vi "Read u.vi"(8 "error in (no error)":errorcluster, 11 "tCRD Data in":refnum<class "tCRD Data.lvclass">) -> (0 "error out":errorcluster, 2 "u":sgl, 3 "tCRD Data out":refnum<class "tCRD Data.lvclass">)   [LabVIEW 2013, in "tCRD Data.lvclass"]
uses:
  tCRD Data.lvclass
  tCRD Data.lvclass/tCRD Data.ctl
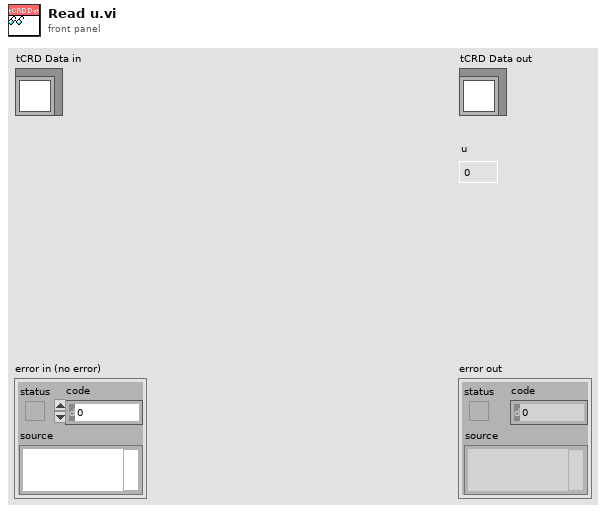
[diagram p1: front panel]
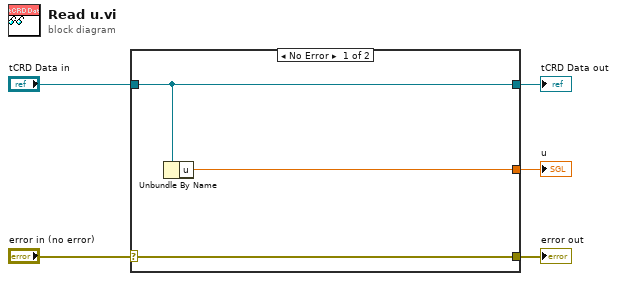
[diagram p0: block diagram]
diagram:
  n1 = case shown="No Error" "error in (no error)" {
    selector: "error in (no error)" -> [w8 w9]
    tunnel: [w8 w9] -> w4
    tunnel: [w7 w10] -> w2
    tunnel: "tCRD Data in" -> [w7 w10]
    tunnel: [w6 _] -> w1
    frame No Error {
      n2 = Unbundle By Name(w7) -> ("u"=w6:sgl)
    }
    frame Error {
    }
  }
  "error out" <- w4
  "tCRD Data out" <- w2
  "u" <- w1
